vi "Get PCL Decimation.vi"(8 "error in (no error)":errorcluster, 11 "instrument addon refnum in":T1 format="%.0x") -> (0 "error out":errorcluster, 2 "PCL decimation":u32, 3 "instrument addon refnum out":T1=18446744073709551615 format="%.0x")   [LabVIEW 2020, in "Instrument Addon Scripting API.lvlib"]
doc: "Returns the PCL decimation value of the specified Instrument Addon Custom Device."
uses:
  Instrument Addon Scripting API.lvlib
  <vilib>/NI VeriStand/Custom Device API/Custom Device Item Ref.ctl
  Shared Directory/Constants.vi
  Dependencies.llb/Instrument_Addon_Scripting_Dependencies_SysDef.Property.Get.U32.vi
  Dependencies.llb/Instrument_Addon_Scripting_Dependencies_Advanced System Definition.lvlib
  Shared Directory/Instrument Addon Shared.lvlib
  <vilib>/NI VeriStand/Custom Device API/Custom Device API.lvlib
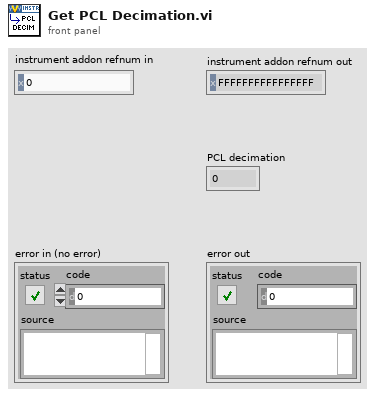
[diagram p1: front panel]
types:
  T1 = typedef "Custom Device API.lvlib/Custom Device Item Ref.ctl" = u64
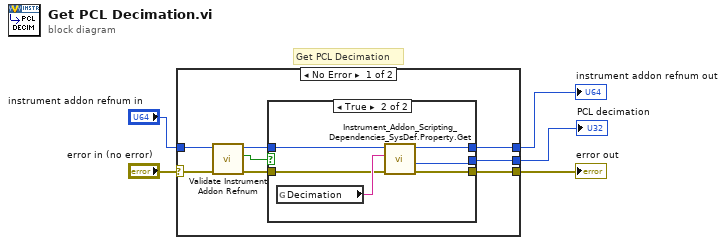
[diagram p0: block diagram]
diagram:
  # "Get PCL Decimation"
  n1 = case shown="No Error" "error in (no error)" {
    selector: "error in (no error)" -> [w13 w23]
    tunnel: "instrument addon refnum in" -> [w11 w22]
    tunnel: [w8 _] -> w4
    tunnel: [w9 w23] -> w3
    tunnel: [w7 w22] -> w1
    frame No Error {
      n2 = call "Validate Instrument Addon Refnum.vi"("Error In"=w13, "Refnum In"=w11) -> ("Error Out"=w12:errorcluster, "Is Instrument Addon?"=w10:bool, "Refnum Out"=w6:T1)  [unwired: 7 in]
      n3 = case shown="True" w10 {
        tunnel: w12 -> [w15 w16]
        tunnel: [w15 w20] -> w9
        tunnel: [_ w19] -> w8
        tunnel: [w14 w18] -> w7
        tunnel: w6 -> [w14 w17]
        frame False {
        }
        frame True {
          n4 = global read "Constants.vi" "Decimation"() -> (w21:string)
          n5 = call-poly "Instrument_Addon_Scripting_Dependencies_SysDef.Property.Get.vi"("error in (no error)"=w16, "Property Name"=w21, "nodeID"=w17) -> ("error out"=w20:errorcluster, "Value out"=w19:u32, "nodeID out"=w18:u64)  [unwired: 5 in, 1 out]
        }
      }
    }
    frame Error {
    }
  }
  "PCL decimation" <- w4
  "error out" <- w3
  "instrument addon refnum out" <- w1
